vi "IC_SetPhysicalExposure.vi"(1 "Exposure":i32, 2 "ICImagingControl 2":refnum<k7>) -> (0 "ICImagingControl":refnum<k7>)   [LabVIEW 2020]
doc: "This VI tries to set the Physical Values Exposure value. The Physical Values is defines the exposure time as 2^n = secons, e.g -6 = 2^-6 = 1/64 seconds."
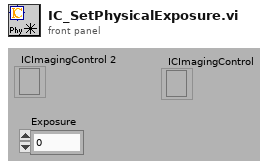
[diagram p1: front panel]
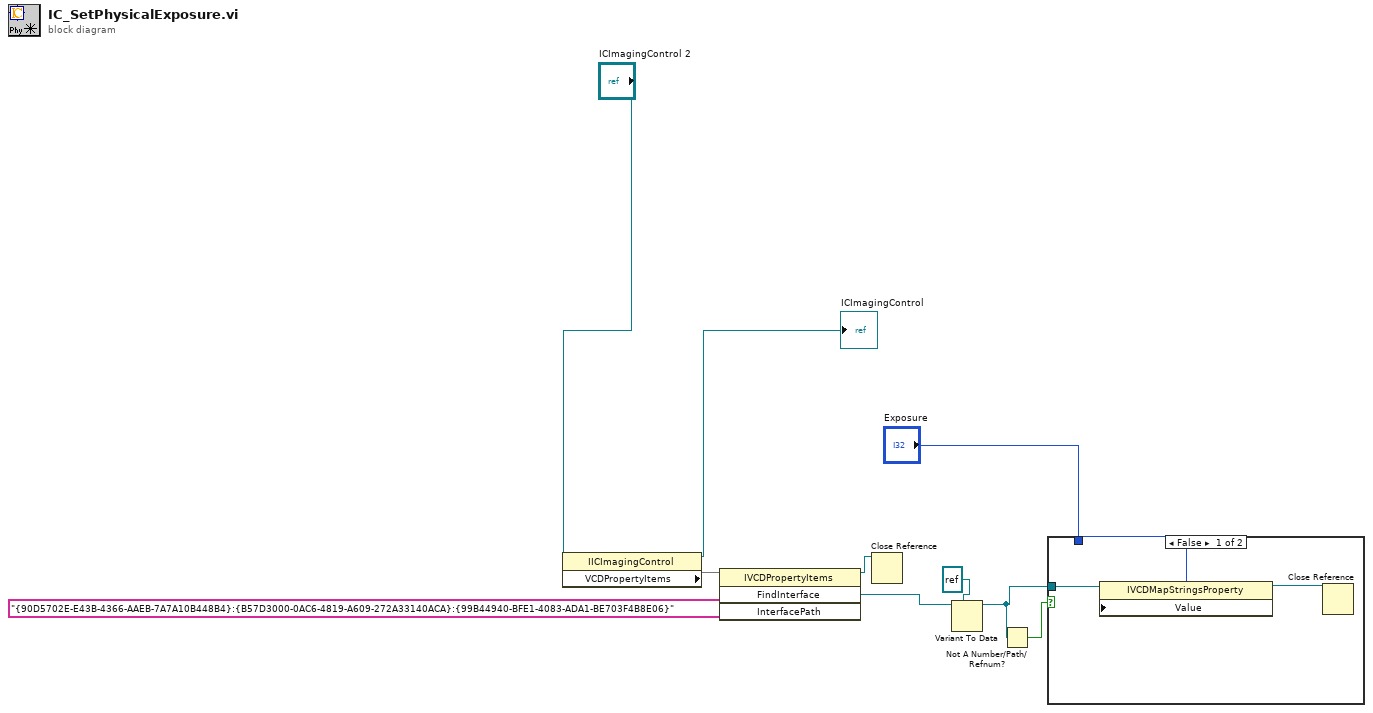
[diagram p0: block diagram]
diagram:
  n1 = property class="IICImagingControl"(reference="ICImagingControl 2") -> (reference out=→"ICImagingControl":refnum<k7>, "VCDPropertyItems"=w7)  [unwired: 1 in, 1 out]
  n2 = invoke class="IVCDPropertyItems" method="FindInterface"(reference=w7, "InterfacePath"="{90D5702E-E43B-4366-AAEB-7A7A10B448B4}:{B57D3000-0AC6-4819-A609-272A33140ACA}:{99B44940-BFE1-4083-ADA1-BE703F4B8E06}" ("ElementPath")) -> (reference out=w3:refnum<k7>, "FindInterface"=w4:refnum<k7>)  [unwired: 2 in, 2 out]
  n3 = Close Reference(reference=w3) -> ()  [unwired: 1 in, 1 out]
  n4 = Variant To Data(type=refnum<k7> refnum ("ICImagingControl3.IVCDMapStringsProperty"), Variant=w4) -> (data=w2:refnum<k7>)  [unwired: 1 in, 1 out]
  n5 = Not A Number/Path/Refnum?(number/path/refnum=w2) -> (NaN/Path/Refnum?=w1:bool)
  n6 = case shown="False" w1 {
    tunnel: w2 -> [w12 _]
    tunnel: "Exposure" -> [w11 _]
    frame False {
      n7 = property class="IVCDMapStringsProperty"(reference=w12, "Value"=w11) -> (reference out=w13:refnum<k7>)  [unwired: 1 in, 1 out]
      n8 = Close Reference(reference=w13) -> ()  [unwired: 1 in, 1 out]
    }
    frame True {
    }
  }
